vi "Get.vi"(8 "error in (no error)":errorcluster, 11 "Simulator in":refnum<class "Simulator.lvclass">) -> (0 "error out":errorcluster, 2 "Numeric":dbl, 3 "Simulator out":refnum<class "Simulator.lvclass">)   [LabVIEW 2018, in "Simulator.lvclass"]
uses:
  Simulator.lvclass
  Simulator.lvclass/Simulator.ctl
  Instrument/Instrument.lvclass
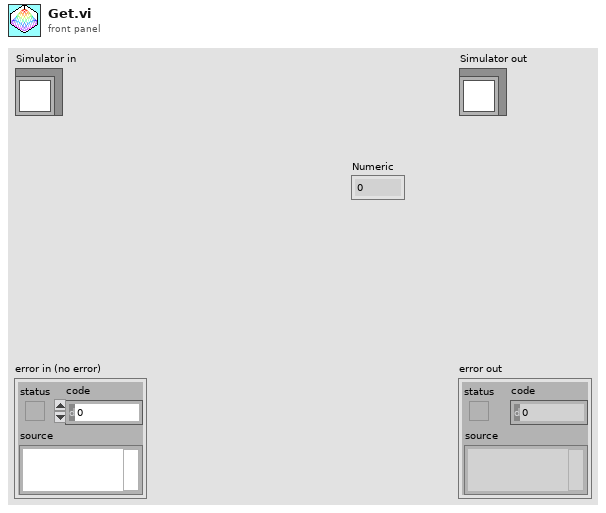
[diagram p1: front panel]
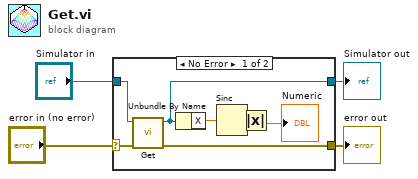
[diagram p0: block diagram]
diagram:
  n1 = case shown="No Error" "error in (no error)" {
    selector: "error in (no error)" -> [w9 w12]
    tunnel: [w11 w12] -> w4
    tunnel: [w8 w13] -> w3
    tunnel: "Simulator in" -> [w10 w13]
    frame No Error {
      n2 = call-parent "Get.vi"("error in (no error)"=w9, "Instrument in"=w10) -> ("error out"=w11:errorcluster, "Instrument out"=w8:refnum<class "Simulator.lvclass">)  [unwired: 7 in, 1 out]
      n3 = Unbundle By Name(w8) -> ("X"=w7:dbl)
      n4 = Sinc(1:w7) -> (0:w6:dbl)
      n5 = Absolute Value(x=w6) -> (abs(x)=→"Numeric":dbl)
    }
    frame Error {
    }
  }
  "error out" <- w4
  "Simulator out" <- w3
